vi "INI Read write string.vi"(5 "key":string, 6 "read/write raw string? (F)":bool, 7 "section":string, 8 "error in":errorcluster, 9 "Default":string, 10 "string in":string, 11 "Read|Write":T1) -> (0 "error out":errorcluster, 2 "string out":string)   [LabVIEW 2013]
doc: "This .vi reads/writes a string to the config file. During Write, \"string in\" is passed to \"string out\""
uses:
  Read write mode.ctl
  <vilib>/Utility/config.llb/Read Key (String).vi
  <vilib>/Utility/config.llb/Write Key (String).vi
  <vilib>/Utility/config.llb/NI_LVConfig.lvlib
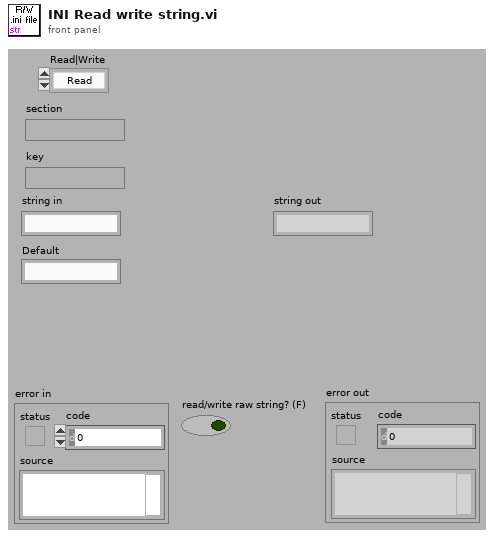
[diagram p1: front panel]
types:
  T1 = typedef "Read write mode.ctl" = enum16{"Read", "Write"}
  T2 = typedef "Semaphore RefNum" = refnum<k1>
  T3 = typedef "NI_LVConfig.lvlib/Config Data RefNum.ctl" = refnum<k1>
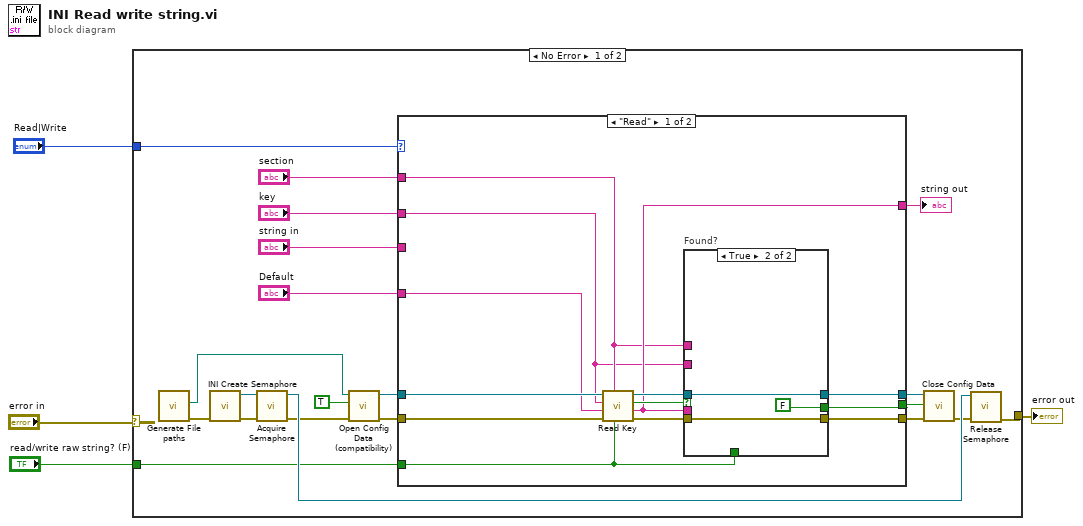
[diagram p0: block diagram]
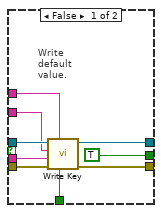
[diagram p2: hidden frame]
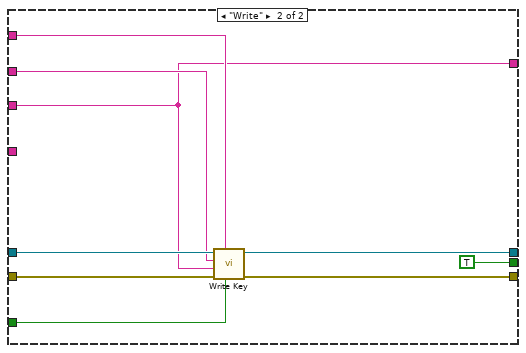
[diagram p3: hidden frame]
diagram:
  n1 = case shown="No Error" "error in" {
    selector: "error in" -> [_ w60]
    tunnel: "Read|Write" -> [w25 _]
    tunnel: [w10 w60] -> w2
    tunnel: "read/write raw string? (F)" -> [w7 _]
    frame No Error {
      n2 = call "Generate File paths.vi"() -> ("error out"=w6:errorcluster, ".ini path"=w5:path)  [unwired: 1 in, 9 out]
      n3 = call "INI Create Semaphore.vi"("error in"=w6) -> ("error out"=w9:errorcluster, "semaphore"=w8:T2)  [unwired: 1 in, 4 out]
      n4 = call <vilib>:"Acquire Semaphore.vi"("error in (no error)"=w9, "semaphore"=w8) -> ("error out"=w12:errorcluster, "semaphore out"=w13:T2)  [unwired: 1 in, 3 out]
      n5 = call <vilib>:"Open Config Data (compatibility).vi"("error in (no error)"=w12, "create file if necessary (T)"=TRUE ("create file if necessary? (T)"), "configuration file path"=w5) -> ("error out"=w20:errorcluster, "refnum"=w23:T3)  [unwired: 6 in, 1 out]
      n6 = case shown="\"Read\"" w25 {
        tunnel: [w29 w58] -> w22
        tunnel: w23 -> [w38 w59]
        tunnel: [w28 w57] -> w21
        tunnel: w20 -> [w37 w56]
        tunnel: "section" -> [w31 w55]
        tunnel: "key" -> [w30 w54]
        tunnel: [w32 w52] -> w17
        tunnel: "string in" -> [_ w52]
        tunnel: [w26 TRUE ("write configuration file? (T)")] -> w15
        tunnel: "Default" -> [w36 _]
        tunnel: w7 -> [w27 w51]
        frame "Read" {
          n7 = call-poly <vilib>:"Read Key.vi"("read raw string? (F)"=w27, "section"=w31, "error in (no error)"=w37, "default value"=w36, "key"=w30, "refnum"=w38) -> ("error out"=w34:errorcluster, "value"=w32:string, "found?"=w35:bool, "refnum out"=w33:T3)  [unwired: 2 out]
          n8 = case "Found?" shown="True" w35 {
            tunnel: w34 -> [w47 w50]
            tunnel: [w46 w50] -> w29
            tunnel: w32 -> [w45 _]
            tunnel: w33 -> [w44 w49]
            tunnel: [w43 w49] -> w28
            tunnel: w31 -> [w42 _]
            tunnel: w30 -> [w41 _]
            tunnel: w27 -> [w40 _]
            tunnel: [TRUE ("write configuration file? (T)") FALSE ("write configuration file? (T)")] -> w26
            frame False {
              # "Write\ndefault\nvalue."
              n9 = call-poly <vilib>:"Write Key.vi"("write raw string? (F)"=w40, "section"=w42, "error in (no error)"=w47, "value"=w45, "key"=w41, "refnum"=w44) -> ("error out"=w46:errorcluster, "refnum out"=w43:T3)  [unwired: 4 out]
            }
            frame True {
            }
          }
        }
        frame "Write" {
          n10 = call-poly <vilib>:"Write Key.vi"("write raw string? (F)"=w51, "section"=w55, "error in (no error)"=w56, "value"=w52, "key"=w54, "refnum"=w59) -> ("error out"=w58:errorcluster, "refnum out"=w57:T3)  [unwired: 4 out]
        }
      }
      "string out" <- w17
      n11 = call <vilib>:"Close Config Data.vi"("error in (no error)"=w22, "write file if changed (T)"=w15, "refnum"=w21) -> ("error out"=w11:errorcluster)  [unwired: 8 out]
      n12 = call <vilib>:"Release Semaphore.vi"("error in (no error)"=w11, "semaphore"=w13) -> ("error out"=w10:errorcluster)  [unwired: 5 out]
    }
    frame Error {
    }
  }
  "error out" <- w2
